vi "Write Topics List.vi"(8 "error in (no error)":errorcluster, 10 "Topics List":string[](array[string]), 11 "SelectTopics in":refnum<class "SelectTopics.lvclass">) -> (0 "error out":errorcluster, 3 "SelectTopics out":refnum<class "SelectTopics.lvclass">)   [LabVIEW 2023, in "uLib.lvlib" / "SelectTopics.lvclass"]
uses:
  SelectTopics.lvclass
  SelectTopics.lvclass/SelectTopics.ctl
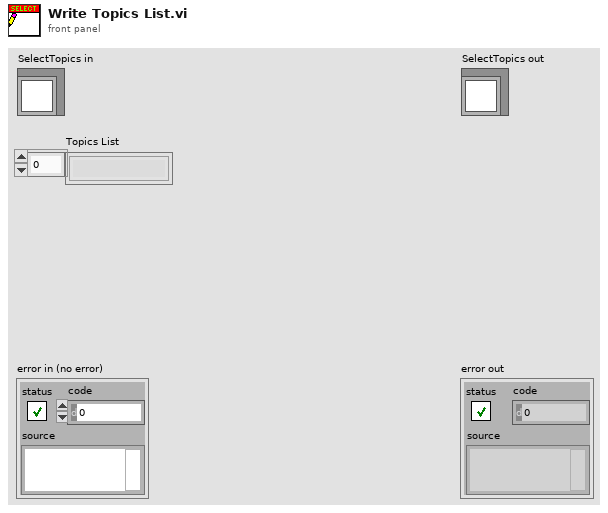
[diagram p1: front panel]
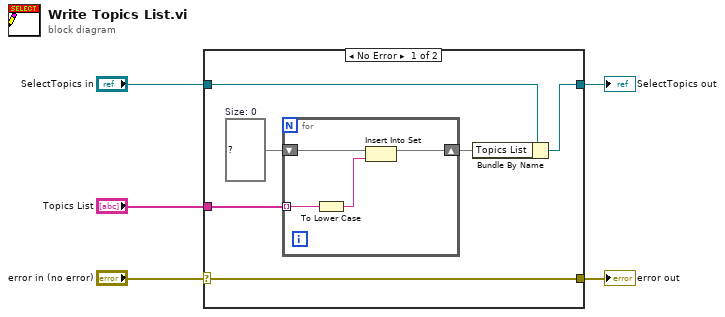
[diagram p0: block diagram]
diagram:
  n1 = case shown="No Error" "error in (no error)" {
    selector: "error in (no error)" -> [w11 w16]
    tunnel: [w11 w16] -> w4
    tunnel: [w9 w17] -> w2
    tunnel: "SelectTopics in" -> [w10 w17]
    tunnel: "Topics List" -> [w6 _]
    frame No Error {
      w8 = set{string} {}  # Size: 0
      n2 = for {
        tunnel: w6 -> [w15] mode=indexing
        shift-right: [w13] -> w7
        shift-left: w8 -> [w12]
        n3 = To Lower Case(string=w15) -> (all lower case string=w14:string)
        n4 = Insert Into Set(10:w14, 11:w12) -> (3:w13:set{string})  [unwired: 1 out]
      }
      n5 = Bundle By Name(cluster=w10, "Topics List"=w7) -> (w9:refnum<class "SelectTopics.lvclass">)
    }
    frame Error {
    }
  }
  "error out" <- w4
  "SelectTopics out" <- w2
